vi "Get Primary Direction Array.vi"(3 "Primary Direction":T1) -> (1 "Direction Array":T1[](array[typedef])=[enum."NW", enum."N", enum."NE", enum."E", enum."SE", enum."S", enum."SW", enum."W"])   [LabVIEW 2020, in "AntFarm_MB.lvclass"]
uses:
  AntFarm_MB.lvclass
  Type Defs/Direction Enum.ctl
  TypeDefs/ENUM_New Direction Select.ctl
  Type Defs/SB Type Defs.lvlib
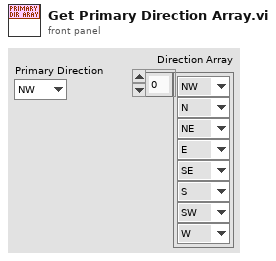
[diagram p1: front panel]
types:
  T1 = typedef "SB Type Defs.lvlib/Direction Enum.ctl" = enum16{"NW", "N", "NE", "E", "SE", "S", "SW", "W"}
  T2 = typedef "ENUM_New Direction Select.ctl" = enum16{"Same", "CCW 45", "CW 45", "CCW 90", "CW 90", "CCW 135", "CW 135", "Opposite"}
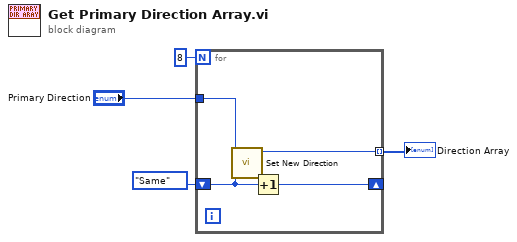
[diagram p0: block diagram]
diagram:
  n1 = for {
    N: 8 -> [_]
    shift-right: [w7] -> _
    shift-left: ENUM_New_Direction_Select."Same" ("New Direction") -> [w8]
    tunnel: "Primary Direction" -> [w6]
    tunnel: [w5] -> w1 mode=indexing
    n2 = call "Set New Direction.vi"("New Direction"=w8, "Target Direction in"=w6) -> ("Target Direction out"=w5:T1)  [unwired: 9 in]
    n3 = Increment(x=w8) -> (x+1=w7:T2)
  }
  "Direction Array" <- w1
